vi "FTW-Ether-Instance.vi"() -> ()   [LabVIEW 2012, in "FTW-Actor.lvlib" / "FTW-Ether.lvclass"]
uses:
  FTW-Ether.lvclass
  EventLogger/FTW-Logger.lvclass
  Utility/FTW-Actor-Address.ctl
  FTW-Actor.lvlib
panel:
  in  "Application Version":string
  in  "Application Name":string
  in  "Logger Address":T1
  in  "Default Linger":i32=100 format="%dmsec"
  in  "ØMQ Context":u64 format="%016x"
  in  "Logger":refnum<class "FTW-Logger.lvclass">
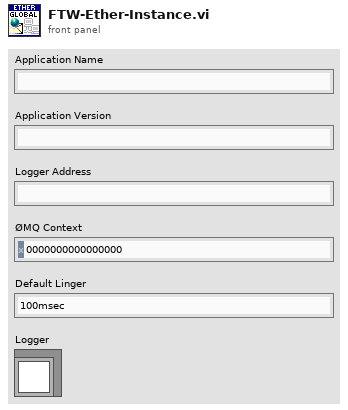
[diagram p1: front panel]
types:
  T1 = typedef "FTW-Actor.lvlib/FTW-Actor-Address.ctl" = string
diagram:
